vi "Teleop.vi"(10 "Match Info":T1={"Autonomous Elapsed Seconds"=0.0, "TeleOp Elapsed Seconds"=0.0, "Disabled Elapsed Seconds"=0.0, "Visited Autonomous"=FALSE, "Visited TeleOp"=FALSE, "Visited Disabled"=FALSE, "Autonomous Settings"={"Autonomous Style"=enum."Independent", "VI Refnum"=refnum}}, 11 "Call Context":T2) -> ()   [LabVIEW 2017]
doc: "This VI is called for each TeleOp packet received from the DS where the robot is not disabled. It is often used to read from the joysticks and update I/O or to update setpoints for timed control loops. It should complete and return within 20 milliseconds or it may miss DS packets."
uses:
  <vilib>/Rock Robotics/WPI/DriverStation/WPI_DriverStationDerivedRobotMode.ctl
  <vilib>/Rock Robotics/WPI/DriverStation/WPI_DriverStationMatch Info.ctl
  Drive/Drive Notifier.ctl
  Drive/Drive Control Type.ctl
  Intake/Intake Notifier.ctl
  Intake/Intake Control Type.ctl
  Lift/Lift Notifier.ctl
  Lift/Lift Control Type.ctl
  Lift/Lift Enum States.ctl
  RPED/RPED Notifier.ctl
  RPED/RPED Control Type.ctl
  Intake Rotation/Intake Rotation Notifier.ctl
  Intake Rotation/Intake Rotation Control Type.ctl
  Intake Rotation/Arm Enum States.ctl
  LEDs/LED Notifier.ctl
  LEDs/LED Control Type.ctl
  <vilib>/Rock Robotics/Network Tables/NT Write String.vi
  Drive/Drive Globals.vi
  Lift/Lift Globals.vi
  Intake/Intake Globals.vi
  RPED/RPED Globals.vi
  Intake Rotation/Intake Rotation Globals.vi
  LEDs/LED Globals.vi
  Utility VIs/Refnum Names.vi
  <vilib>/Rock Robotics/WPI/Utilities/WPI_GetSetVariantRefNum.vi
  Robot Global Data.vi
panel:
  out "Visited Disabled":bool
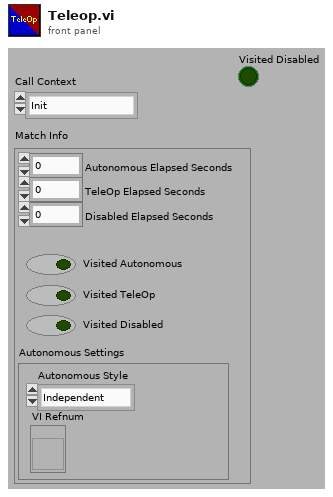
[diagram p1: front panel]
types:
  T1 = typedef "WPI_DriverStationMatch Info.ctl" = cluster{"Autonomous Elapsed Seconds":dbl, "TeleOp Elapsed Seconds":dbl, "Disabled Elapsed Seconds":dbl, "Visited Autonomous":bool, "Visited TeleOp":bool, "Visited Disabled":bool, "Autonomous Settings":cluster{"Autonomous Style":enum16{"Iterative", "Independent"}, "VI Refnum":refnum<vi>}}
  T2 = typedef "WPI_DriverStationDerivedRobotMode.ctl" = enum16{"Init", "Execute", "Stop"}
  T3 = typedef "LED Notifier.ctl" = cluster{"LED Control Type":T4, "Climbing":bool, "Auto Tracking":bool, "Ready for Cube Floor":bool, "Ready for Cube Portal":bool}
  T4 = typedef "LED Control Type.ctl" = enum16{"Off", "Waiting On Field", "Connected ", "Cube In Intake", "Climbing", "Auto Cube Capture", "Ready for Cube Floor", "Ready for Cube Portal"}
  T5 = typedef "Intake Rotation Notifier.ctl" = cluster{"Step":i32, "Intake Rotation Control Type":T6, "Parameter 1":dbl, "Parameter 2":dbl, "Intake Rotation Notifier":refnum<notifier>, "Manual Up":bool, "Manual Down":bool, "Climb":bool, "Switch":bool, "Scale Low":bool, "Scale High":bool, "Stow":bool, "Load":bool, "Scale Mid":bool, "Exchange":bool, "Set Position":T7, "Portal":bool}
  T6 = typedef "Intake Rotation Control Type.ctl" = enum16{"No Op", "Manual Up", "Position", "Manual Down", "PositionAuto"}
  T7 = typedef "Arm Enum States.ctl" = enum16{"Current Position", "Climb", "Load", "Portal", "Switch", "Scale High", "Scale Mid", "Scale Low", "Exchange", "Stow"}
  T8 = typedef "RPED Notifier.ctl" = cluster{"RPED Control Type":T9, "Step":i32, "Left Forward":bool, "Right Forward":bool, "Parameter 1":dbl, "Parameter 2":dbl, "Parameter 3":dbl, "RPED Notifier":refnum<notifier>, "Left Back":bool, "Right Back":bool, "Right":bool, "Left":bool}
  T9 = typedef "RPED Control Type.ctl" = enum16{"No Op", "Left Manual", "Right Manual", "Time", "Left", "Right", "Left_Slow", "Right_Slow", "Left_Distance", "Right_Distance"}
  T10 = typedef "Lift Notifier.ctl" = cluster{"Lift Control Type":T11, "Step":i32, "Set Position":T12, "Climb":bool, "Switch":bool, "Scale Low":bool, "Scale Mid":bool, "Scale High":bool, "Stow":bool, "Load":bool, "Climb Actuation":bool, "Manual Up":bool, "Manual Down":bool, "Parameter 1":dbl, "Parameter 2":dbl, "Parameter 3":dbl, "Lift Notifier":refnum<notifier>, "Exchange":bool, "Brake":bool, "Portal":bool}
  T11 = typedef "Lift Control Type.ctl" = enum16{"No Op", "Position", "Climb Actuation", "Manual Up", "Manual Down", "PositionAuto", "Position_kP", "Position_Delay"}
  T12 = typedef "Lift Enum States.ctl" = enum16{"Climb", "Load", "Portal", "Switch", "Scale High", "Scale Mid", "Scale Low", "Exchange", "Stow", "Current Position"}
  T13 = typedef "Intake Notifier.ctl" = cluster{"Intake Control Type":T14, "Step":i32, "In":bool, "Speed":dbl, "Out":bool, "Parameter 1":dbl, "Parameter 2":dbl, "Intake Notifier":refnum<notifier>, "Actuate Cube":bool, "Speed In":dbl, "Speed Out":dbl, "Load":bool, "Override":bool, "Exchange":bool, "Intake Open":bool}
  T14 = typedef "Intake Control Type.ctl" = enum16{"No Op", "In", "Out", "Test Mode", "Cube_In", "Cube_Out", "State_Change"}
  T15 = typedef "Drive Notifier.ctl" = cluster{"Drive Control Type":T16, "Throttle":dbl, "Twist":dbl, "Step":i32, "High Gear":bool, "Parameter 1":dbl, "Parameter 2":dbl, "Parameter 3":dbl, "Drive Notifier":refnum<notifier>, "AutoTrack":bool}
  T16 = typedef "Drive Control Type.ctl" = enum16{"No_Op", "Basic Drive", "Time", "Heading", "Hybrid_Turn", "RC_Speed", "Switch_Slots", "AutoTrack_Cube", "Speed Test", "Turn_Cube", "To_Cube", "Wait", "Distance_Slow", "Distance", "D_H_Delay", "Distance_Delay", "Heading_Cap", "Heading_Tight", "Cube_Heading", "Distance_Ramp"}
  T17 = typedef "Joystick Controls.ctl" = cluster{"Pilot Left Joystick X":dbl, "Pilot Left Joystick Y":dbl, "Pilot A Button":bool, "Pilot B Button":bool, "Pilot X Button":bool, "Pilot Y Button":bool, "Pilot Left Bumper":bool, "Pilot Right Bumper":bool, "Pilot View Button":bool, "Pilot Menu Button":bool, "Pilot Left Joystick Press":bool, "Pilot Right Joystick Press":bool, "Pilot Left Trigger":dbl, "Pilot Right Joystick X":dbl, "Pilot Right Joystick Y":dbl, "Pilot Right Trigger":dbl, "Copilot Left Joystick X":dbl, "Copilot Left Joystick Y":dbl, "Copilot A Button":bool, "Copilot B Button":bool, "Copilot X Button":bool, "Copilot Y Button":bool, "Copilot Left Bumper":bool, "Copilot Right Bumper":bool, "Copilot View Button":bool, "Copilot Menu Button":bool, "Copilot Left Joystick Press":bool, "Copilot Right Joystick Press":bool, "Copilot Left Trigger":dbl, "Copilot Right Joystick X":dbl, "Copilot Right Joystick Y":dbl, "Copilot Right Trigger":dbl, "Pilot D-Pad":i16, "Copilot D-Pad":i16}
  T18 = typedef "WPI_CompressorDevRef.ctl" = cluster{"DevStatus":errorcluster, "Pneumatics Control Module":u8}
  T19 = cluster{"offsetAngle H":dbl, "offsetAngle V":dbl, "area":dbl, "skew":dbl}
  T20 = typedef "WPI_JoystickDevRef.ctl" = cluster{"Device":T21}
  T21 = typedef "WPI_JoystickDeviceEnum.ctl" = enum16{"USB 0", "USB 1", "USB 2", "USB 3", "USB 4", "USB 5"}
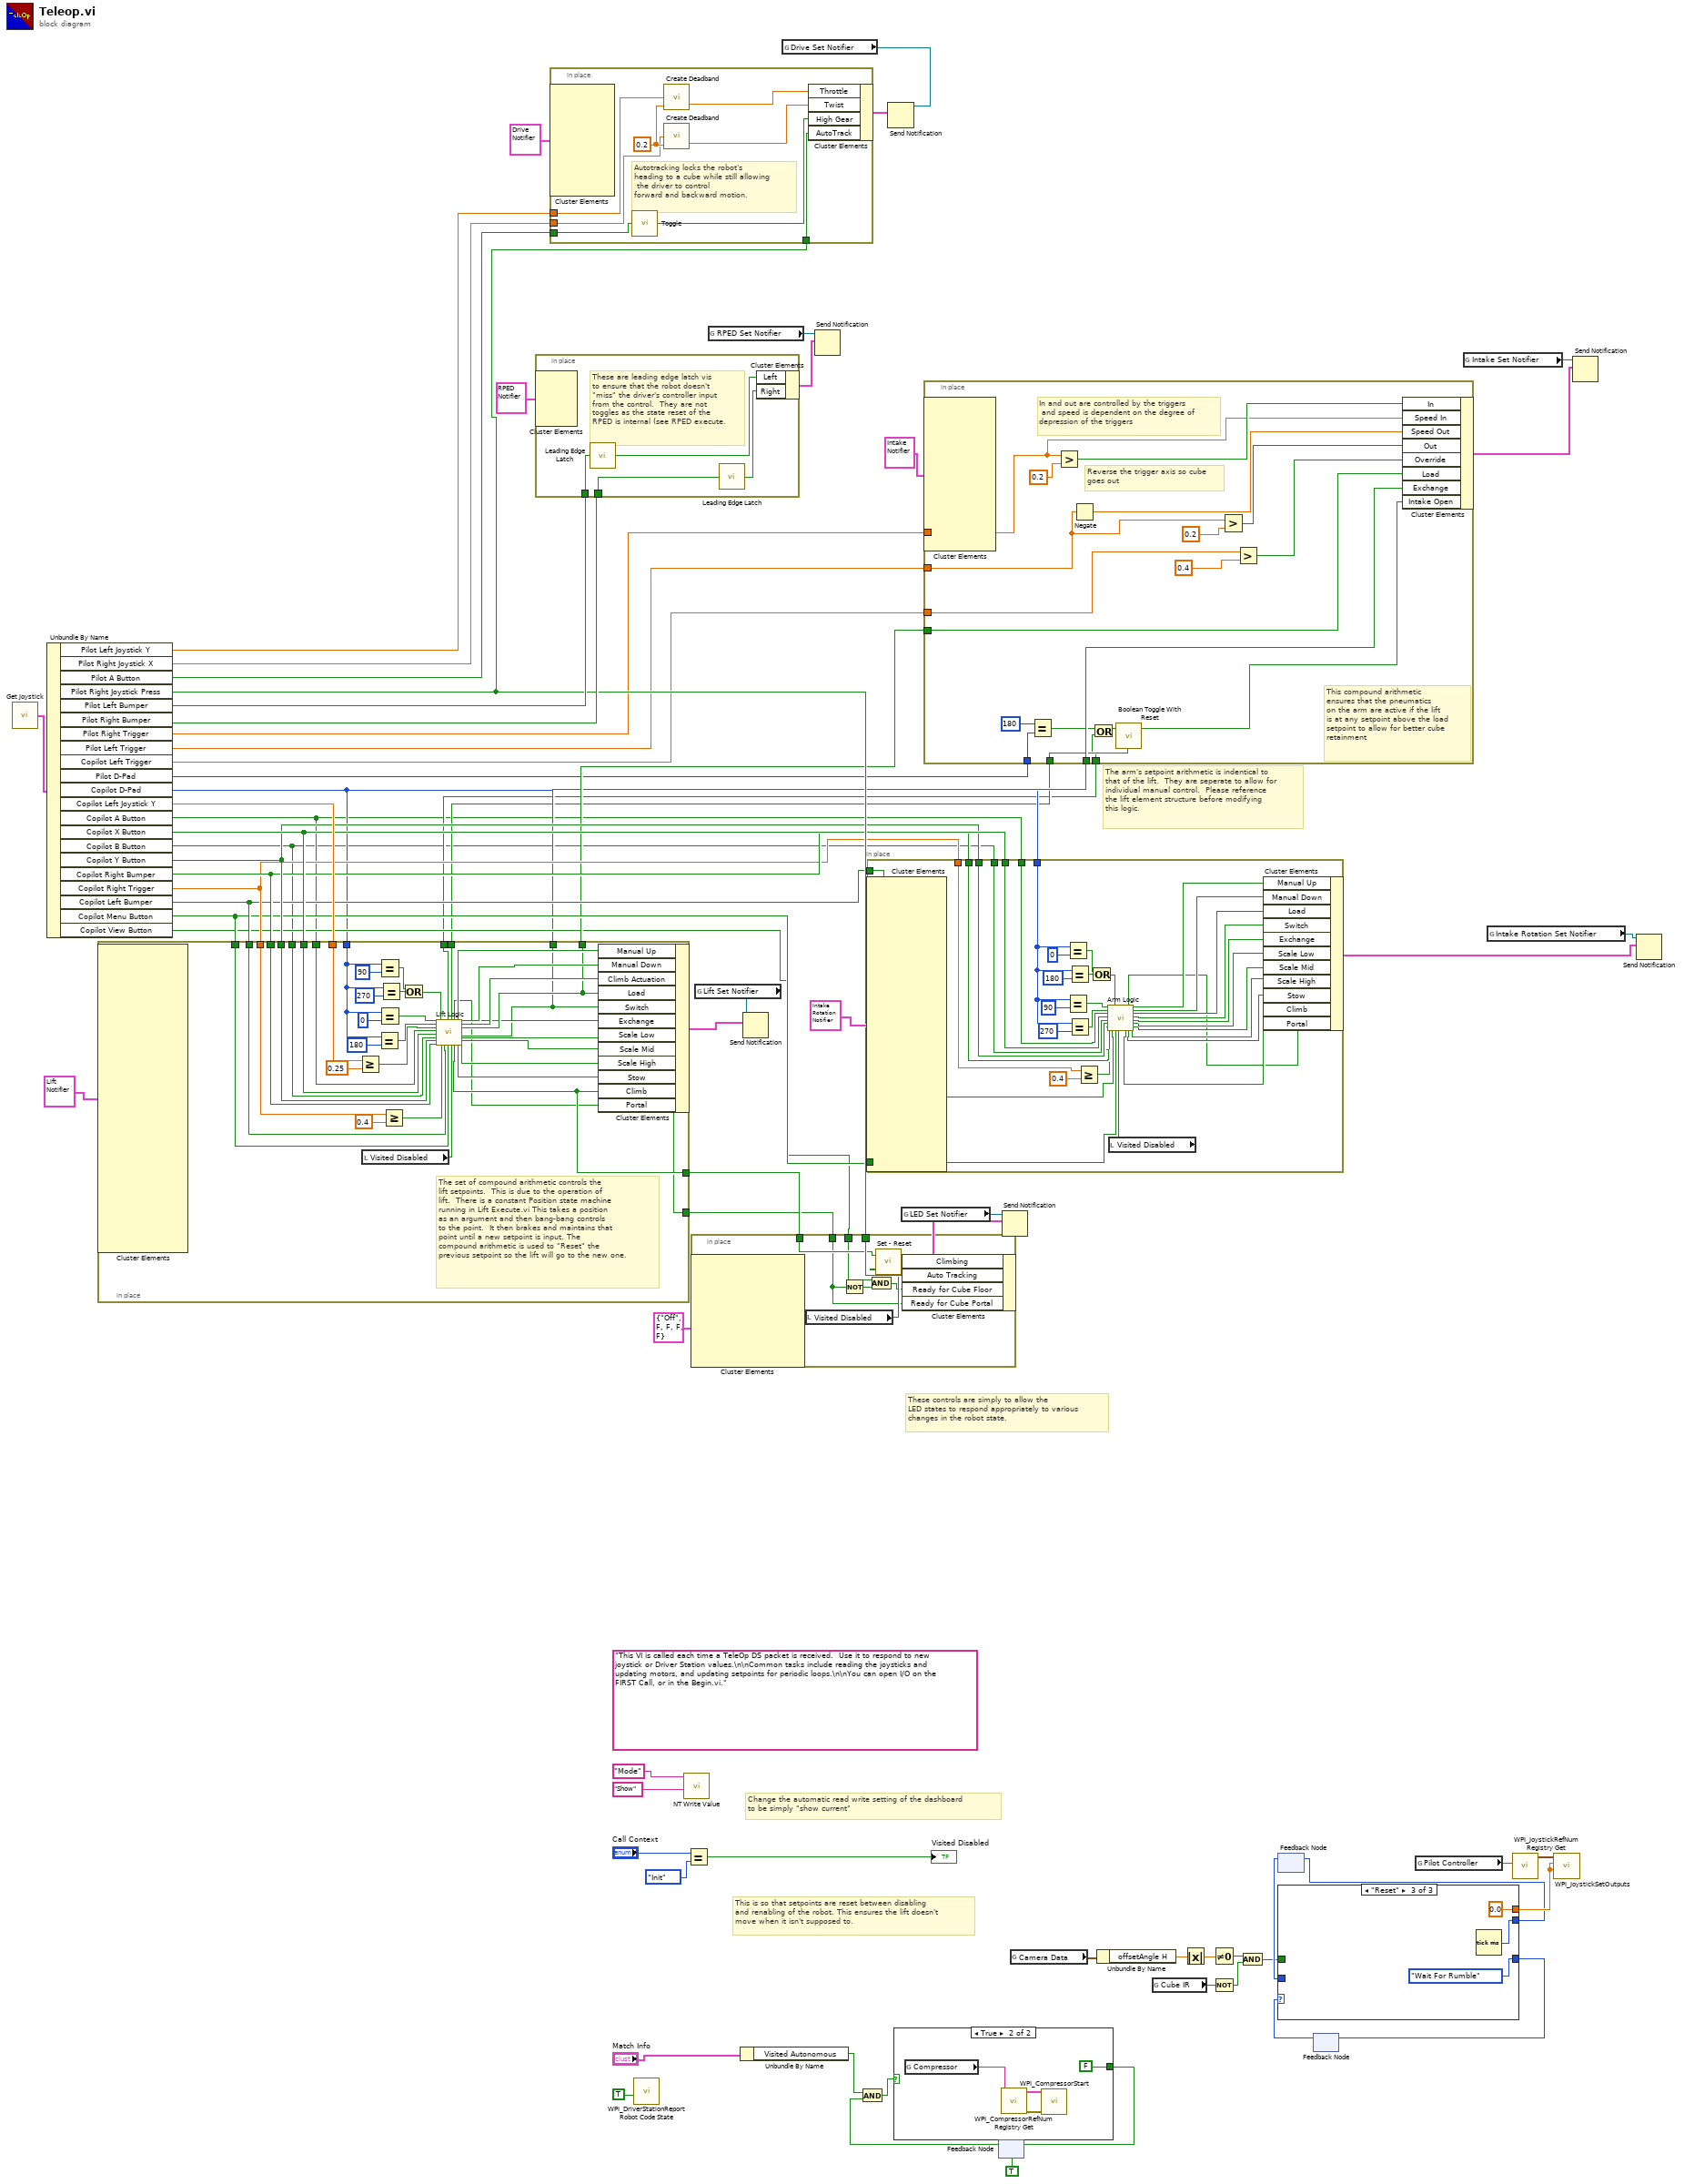
[diagram p0: block diagram]
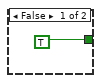
[diagram p2: hidden frame]
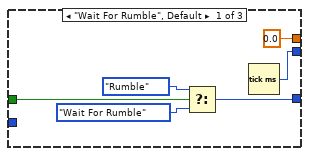
[diagram p3: hidden frame]
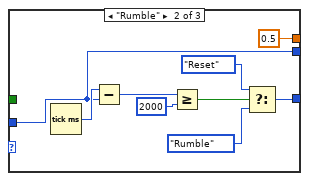
[diagram p4: hidden frame]
diagram:
  (unwired) "This VI is called each time a TeleOp DS packet is received.  Use it to respond to new joystick or Driver Station values.\n\nCommon tasks include reading the joysticks and updating motors, and updating setpoints for periodic loops.\n\nYou can open I/O on the FIRST Call, or in the Begin.vi."
  # "The arm's setpoint arithmetic is indentical to \nthat of the lift.  They are seperate to allow for\nindividual manual control.  Please reference \nthe lift element structure before modifying\nthis logic."
  # "Change the automatic read write setting of the dashboard\nto be simply \"show current\""
  # "This is so that setpoints are reset between disabling\nand renabling of the robot. This ensures the lift doesn't\nmove when it isn't supposed to."
  # "These controls are simply to allow the \nLED states to respond appropriately to various\nchanges in the robot state."
  n1 = call "Get Joystick.vi"() -> ("Joystick Controls"=w71:T17)  [unwired: 7 in]
  n2 = Unbundle By Name(w71) -> ("Pilot Left Joystick Y"=w39:dbl, "Pilot Right Joystick X"=w36:dbl, "Pilot A Button"=w35:bool, "Pilot Right Joystick Press"=w34:bool, "Pilot Left Bumper"=w38:bool, "Pilot Right Bumper"=w37:bool, "Pilot Right Trigger"=w33:dbl, "Pilot Left Trigger"=w32:dbl, "Copilot Left Trigger"=w24:dbl, "Pilot D-Pad"=w6:i16, "Copilot D-Pad"=w7:i16, "Copilot Left Joystick Y"=w31:dbl, "Copilot A Button"=w2:bool, "Copilot X Button"=w30:bool, "Copilot B Button"=w1:bool, "Copilot Y Button"=w29:bool, "Copilot Right Bumper"=w28:bool, "Copilot Right Trigger"=w27:dbl, "Copilot Left Bumper"=w26:bool, "Copilot Menu Button"=w25:bool, "Copilot View Button"=w22:bool)
  n3 = in-place {
    in-place-border: w7 -> [w73]
    in-place-border: w31 -> [w104]
    in-place-border: w2 -> [w102]
    in-place-border: w30 -> [w101]
    in-place-border: w1 -> [w100]
    in-place-border: w29 -> [w99]
    in-place-border: w28 -> [w98]
    in-place-border: w27 -> [w97]
    in-place-border: w26 -> [w85]
    in-place-border: w25 -> [w87]
    in-place-border: [w88] -> w23
    in-place-border: [w86] -> w15
    in-place-border: [w82] -> w14
    in-place-border: [w81] -> w5
    in-place-border: [w80] -> w4
    in-place-border: [w79] -> w3
    # "The set of compound arithmetic controls the \nlift setpoints.  This is due to the operation of \nlift.  There is a constant Position state machine\nrunning in Lift Execute.vi This takes a position\nas an argument and then bang-bang controls\nto the point.  It then brakes and maintains that\npoint until a new setpoint is input. The \ncompound arithmetic is used to \"Reset\" the\nprevious setpoint so the lift will go to the new one."
    n4 = in-place-cluster #1(T10 {"Lift Control Type"=enum."No Op", "Step"=0, "Set Position"=enum."Load", "Climb"=FALSE, "Switch"=FALSE, "Scale Low"=FALSE, "Scale Mid"=FALSE, "Scale High"=FALSE, "Stow"=FALSE, "Load"=FALSE, "Climb Actuation"=FALSE, "Manual Up"=FALSE, "Manual Down"=FALSE, "Parameter 1"=0.0, "Parameter 2"=0.0, "Parameter 3"=0.0, "Lift Notifier"=refnum, "Exchange"=FALSE, "Brake"=FALSE, "Portal"=FALSE} ("Lift Notifier")) -> ()  [unwired: 12 out]
    n5 = Greater Or Equal?(x=w104, y=0.25) -> (x >= y?=w84:bool)
    n6 = local read "Visited Disabled"() -> (w94:bool)
    n7 = Equal?(x=w73, y=i16 180) -> (x = y?=w107:bool)
    n8 = Equal?(x=w73, y=i16 90) -> (x = y?=w77:bool)
    n9 = Equal?(x=w73, y=i16 0) -> (x = y?=w108:bool)
    n10 = Equal?(x=w73, y=i16 270) -> (x = y?=w78:bool)
    n11 = Greater Or Equal?(x=w97, y=0.4) -> (x >= y?=w95:bool)
    n12 = Or(x=w77, y=w78) -> (x .or. y?=w74:bool)
    n13 = call "Lift Logic.vi"("Manual Up"=w108, "Manual Down"=w107, "Climb Actuation"=w84, "Load"=w102, "Switch"=w101, "Exchange"=w100, "Scale Low"=w99, "Scale Mid"=w98, "Reset State Machine"=w74, "Scale High"=w95, "Stow"=w85, "Climb"=w87, "Visited Disabled"=w94) -> ("Open Arms"=w80:bool, "Reset Arm"=w81:bool, "Portal Out"=w79:bool, "Climb Out"=w86:bool, "Manual Up Out"=w93:bool, "Stow Out"=w109:bool, "Manual Down Out"=w92:bool, "Climb Actuation Out"=w110:bool, "Load Out"=w88:bool, "Switch Out"=w83:bool, "Exchange Out"=w82:bool, "Scale Low Out"=w91:bool, "Scale Mid Out"=w90:bool, "Scale High Out"=w89:bool)  [unwired: 1 in]
    n14 = in-place-cluster #1("Manual Up"=w93, "Manual Down"=w92, "Climb Actuation"=w110, "Load"=w88, "Switch"=w83, "Exchange"=w82, "Scale Low"=w91, "Scale Mid"=w90, "Scale High"=w89, "Stow"=w109, "Climb"=w86, "Portal"=w79) -> (w68:T10)
  }
  n15 = in-place {
    in-place-border: w38 -> [w112]
    in-place-border: w37 -> [w111]
    # "These are leading edge latch vis\nto ensure that the robot doesn't\n\"miss\" the driver's controller input\nfrom the control.  They are not\ntoggles as the state reset of the \nRPED is internal (see RPED execute."
    n16 = in-place-cluster #2(T8 {"RPED Control Type"=enum."No Op", "Step"=0, "Left Forward"=FALSE, "Right Forward"=FALSE, "Parameter 1"=0.0, "Parameter 2"=0.0, "Parameter 3"=0.0, "RPED Notifier"=refnum, "Left Back"=FALSE, "Right Back"=FALSE, "Right"=FALSE, "Left"=FALSE} ("RPED Notifier")) -> ()  [unwired: 2 out]
    n17 = call "Leading Edge Latch.vi"("Input"=w112) -> ("Output"=w114:bool)
    n18 = call "Leading Edge Latch.vi"("Input"=w111) -> ("Output"=w113:bool)
    n19 = in-place-cluster #2("Left"=w114, "Right"=w113) -> (w61:T8)
  }
  n20 = in-place {
    in-place-border: w39 -> [w118]
    in-place-border: w36 -> [w117]
    in-place-border: w35 -> [w116]
    in-place-border: w34 -> [w115]
    w119 = 0.2
    # "Autotracking locks the robot's \nheading to a cube while still allowing\n the driver to control \nforward and backward motion."
    n21 = in-place-cluster #3(T15 {"Drive Control Type"=enum."No_Op", "Throttle"=0.0, "Twist"=0.0, "Step"=0, "High Gear"=FALSE, "Parameter 1"=0.0, "Parameter 2"=0.0, "Parameter 3"=0.0, "Drive Notifier"=refnum, "AutoTrack"=FALSE} ("Drive Notifier")) -> ()  [unwired: 4 out]
    n22 = call "Toggle.vi"("Boolean"=w116) -> ("Boolean Out"=w122:bool)
    n23 = call "Create Deadband.vi"("Input Deadband"=w119, "Input"=w118) -> ("Output"=w121:dbl)  [unwired: 2 in]
    n24 = call "Create Deadband.vi"("Input Deadband"=w119, "Input"=w117) -> ("Output"=w120:dbl)  [unwired: 2 in]
    n25 = in-place-cluster #3("Throttle"=w121, "Twist"=w120, "High Gear"=w122, "AutoTrack"=w115) -> (w70:T15)
  }
  n26 = call <vilib>:"WPI_DriverStationReport Robot Code State.vi"("TeleOp"=TRUE ("Autonomous")) -> ()  [unwired: 10 in, 1 out]
  n27 = call-poly <vilib>:"NT Write Value.vi"("String"="Show", "Name"="Mode") -> ()  [unwired: 9 in, 1 out]
  n28 = Equal?(x="Call Context", y=WPI_DriverStationDerivedRobotMode."Init") -> (x = y?=→"Visited Disabled":bool)
  n29 = in-place {
    in-place-border: w34 -> [w130]
    in-place-border: w22 -> [w125]
    in-place-border: w15 -> [w129]
    in-place-border: w3 -> [w123]
    n30 = in-place-cluster #4(T3 {"LED Control Type"=enum."Off", "Climbing"=FALSE, "Auto Tracking"=FALSE, "Ready for Cube Floor"=FALSE, "Ready for Cube Portal"=FALSE} ("LED Notifier")) -> ()  [unwired: 4 out]
    n31 = local read "Visited Disabled"() -> (w127:bool)
    n32 = Not(x=w123) -> (.not. x?=w124:bool)
    n33 = And(x=w125, y=w124) -> (x .and. y?=w126:bool)
    n34 = call "Set - Reset.vi"("Reset"=w127, "Set"=w129) -> ("Output"=w128:bool)
    n35 = in-place-cluster #4("Climbing"=w128, "Auto Tracking"=w130, "Ready for Cube Floor"=w126, "Ready for Cube Portal"=w123) -> (w52:T3)
  }
  n36 = global read "Lift Globals.vi" "Lift Set Notifier"() -> (w64:refnum<notifier>)
  n37 = global read "RPED Globals.vi" "RPED Set Notifier"() -> (w59:refnum<notifier>)
  n38 = Unbundle By Name("Match Info") -> ("Visited Autonomous"=w11:bool)
  n39 = Send Notification(notification=w68, notifier=w64) -> ()  [unwired: 1 in, 2 out]
  n40 = global read "Drive Globals.vi" "Drive Set Notifier"() -> (w66:refnum<notifier>)
  n41 = Send Notification(notification=w61, notifier=w59) -> ()  [unwired: 1 in, 2 out]
  n42 = in-place {
    in-place-border: w7 -> [w133]
    in-place-border: w2 -> [w148]
    in-place-border: w30 -> [w147]
    in-place-border: w1 -> [w146]
    in-place-border: w29 -> [w145]
    in-place-border: w28 -> [w144]
    in-place-border: w27 -> [w141]
    in-place-border: w26 -> [w140]
    in-place-border: w25 -> [w139]
    n43 = in-place-cluster #5(T5 {"Step"=0, "Intake Rotation Control Type"=enum."No Op", "Parameter 1"=0.0, "Parameter 2"=0.0, "Intake Rotation Notifier"=refnum, "Manual Up"=FALSE, "Manual Down"=FALSE, "Climb"=FALSE, "Switch"=FALSE, "Scale Low"=FALSE, "Scale High"=FALSE, "Stow"=FALSE, "Load"=FALSE, "Scale Mid"=FALSE, "Exchange"=FALSE, "Set Position"=enum."Climb", "Portal"=FALSE} ("Intake Rotation Notifier")) -> ()  [unwired: 11 out]
    n44 = Equal?(x=w133, y=i16 0) -> (x = y?=w132:bool)
    n45 = Equal?(x=w133, y=i16 90) -> (x = y?=w152:bool)
    n46 = Equal?(x=w133, y=i16 180) -> (x = y?=w131:bool)
    n47 = Equal?(x=w133, y=i16 270) -> (x = y?=w151:bool)
    n48 = Greater Or Equal?(x=w141, y=0.4) -> (x >= y?=w142:bool)
    n49 = Or(x=w132, y=w131) -> (x .or. y?=w136:bool)
    n50 = local read "Visited Disabled"() -> (w138:bool)
    n51 = call "Arm Logic.vi"("Manual Up"=w152, "Manual Down"=w151, "Load"=w148, "Switch"=w147, "Exchange"=w146, "Scale Low"=w145, "Scale Mid"=w144, "Scale High"=w142, "Stow"=w140, "Reset State Machine"=w136, "Climb"=w139, "Visited Disabled"=w138) -> ("Climb Out"=w154:bool, "Portal Out"=w137:bool, "Stow Out"=w153:bool, "Manual Up Out"=w162:bool, "Manual Down Out"=w161:bool, "Load Out"=w160:bool, "Switch Out"=w159:bool, "Exchange Out"=w158:bool, "Scale Low Out"=w157:bool, "Scale Mid Out"=w156:bool, "Scale High Out"=w155:bool)  [unwired: 5 in]
    n52 = in-place-cluster #5("Manual Up"=w162, "Manual Down"=w161, "Load"=w160, "Switch"=w159, "Exchange"=w158, "Scale Low"=w157, "Scale Mid"=w156, "Scale High"=w155, "Stow"=w153, "Climb"=w154, "Portal"=w137) -> (w56:T5)
  }
  n53 = Send Notification(notification=w70, notifier=w66) -> ()  [unwired: 1 in, 2 out]
  n54 = global read "LED Globals.vi" "LED Set Notifier"() -> (w50:refnum<notifier>)
  n55 = in-place {
    in-place-border: w33 -> [w176]
    in-place-border: w32 -> [w175]
    in-place-border: w24 -> [w173]
    in-place-border: w23 -> [w171]
    in-place-border: w14 -> [w170]
    in-place-border: w6 -> [w168]
    in-place-border: w5 -> [w166]
    in-place-border: w4 -> [w163]
    # "This compound arithmetic\nensures that the pneumatics\non the arm are active if the lift \nis at any setpoint above the load \nsetpoint to allow for better cube\nretainment"
    # "Reverse the trigger axis so cube\ngoes out"
    # "In and out are controlled by the triggers\n and speed is dependent on the degree of\ndepression of the triggers"
    n56 = in-place-cluster #6(T13 {"Intake Control Type"=enum."No Op", "Step"=0, "In"=FALSE, "Speed"=0.0, "Out"=FALSE, "Parameter 1"=0.0, "Parameter 2"=0.0, "Intake Notifier"=refnum, "Actuate Cube"=FALSE, "Speed In"=0.0, "Speed Out"=0.0, "Load"=FALSE, "Override"=FALSE, "Exchange"=FALSE, "Intake Open"=FALSE} ("Intake Notifier")) -> ()  [unwired: 8 out]
    n57 = Equal?(x=i16 180, y=w168) -> (x = y?=w164:bool)
    n58 = Greater?(x=w176, y=0.2) -> (0:w181:bool)
    n59 = Negate(x=w175) -> (-x=w180:dbl)
    n60 = Or(x=w164, y=w163) -> (x .or. y?=w165:bool)
    n61 = call "Boolean Toggle With Reset.vi"("Input"=w165, "Reset"=w166) -> ("Output"=w167:bool)  [unwired: 25 in]
    n62 = Greater?(x=w175, y=0.2) -> (0:w179:bool)
    n63 = Greater?(x=w173, y=0.4) -> (0:w174:bool)
    n64 = in-place-cluster #6("In"=w181, "Speed In"=w176, "Speed Out"=w180, "Out"=w179, "Override"=w174, "Load"=w171, "Exchange"=w170, "Intake Open"=w167) -> (w69:T13)
  }
  n65 = feedback #7(TRUE) -> (w9:bool)
  n66 = And(x=w11, y=w9) -> (x .and. y?=w12:bool)
  n67 = case shown="True" w12 {
    tunnel: [TRUE FALSE] -> w10
    frame False {
    }
    frame True {
      n68 = global read "Refnum Names.vi" "Compressor"() -> (w186:string)
      n69 = call <vilib>:"WPI_CompressorRefNum Registry Get.vi"("refnum name"=w186) -> ("error out"=w184:errorcluster, "CompressorDevRef"=w185:T18)  [unwired: 9 in]
      n70 = call <vilib>:"WPI_CompressorStart.vi"("error in (no error)"=w184, "CompressorDevRef"=w185) -> ()  [unwired: 8 in, 2 out]
    }
  }
  n71 = feedback-in #7(w10) -> ()
  n72 = Send Notification(notification=w52, notifier=w50) -> ()  [unwired: 1 in, 2 out]
  n73 = global read "Robot Global Data.vi" "Camera Data"() -> (w41:T19)
  n74 = Unbundle By Name(w41) -> ("offsetAngle H"=w40:dbl)
  n75 = global read "Intake Globals.vi" "Cube IR"() -> (w47:bool)
  n76 = Absolute Value(x=w40) -> (abs(x)=w49:dbl)
  n77 = Not Equal To 0?(x=w49) -> (x != 0?=w48:bool)
  n78 = Not(x=w47) -> (.not. x?=w46:bool)
  n79 = And(x=w48, y=w46) -> (x .and. y?=w16:bool)
  n80 = feedback #8() -> (w19:u32)  [unwired: 1 in]
  n81 = feedback #9() -> (w17:enum16{"Wait For Rumble", "Rumble", "Reset"})  [unwired: 1 in]
  n82 = case shown="\"Reset\"" w17 {
    tunnel: [0.0 0.5 0.0] -> w21
    tunnel: [w191 w196 w204] -> w20
    tunnel: w19 -> [_ w196 _]
    tunnel: [w188 w195 enum16{"Wait For Rumble", "Rumble", "Reset"}."Wait For Rumble" ("f")] -> w18
    tunnel: w16 -> [w187 _ _]
    frame "Wait For Rumble", Default {
      n83 = Select(t=enum16{"Wait For Rumble", "Rumble", "Reset"}."Rumble" ("Rumble"), s=w187, f=enum16{"Wait For Rumble", "Rumble", "Reset"}."Wait For Rumble") -> (s? t:f=w188:enum16{"Wait For Rumble", "Rumble", "Reset"})
      n84 = Tick Count (ms)() -> (millisecond timer value=w191:u32)
    }
    frame "Rumble" {
      n85 = Tick Count (ms)() -> (millisecond timer value=w200:u32)
      n86 = Subtract(x=w200, y=w196) -> (x-y=w199:u32)
      n87 = Greater Or Equal?(x=w199, y=u32 2000) -> (x >= y?=w197:bool)
      n88 = Select(t=enum16{"Wait For Rumble", "Rumble", "Reset"}."Reset" ("f"), s=w197, f=enum16{"Wait For Rumble", "Rumble", "Reset"}."Rumble") -> (s? t:f=w195:enum16{"Wait For Rumble", "Rumble", "Reset"})
    }
    frame "Reset" {
      n89 = Tick Count (ms)() -> (millisecond timer value=w204:u32)
    }
  }
  n90 = feedback-in #8(w20) -> ()
  n91 = feedback-in #9(w18) -> ()
  n92 = global read "Refnum Names.vi" "Pilot Controller"() -> (w44:string)
  n93 = global read "Intake Globals.vi" "Intake Set Notifier"() -> (w62:refnum<notifier>)
  n94 = global read "Intake Rotation Globals.vi" "Intake Rotation Set Notifier"() -> (w58:refnum<notifier>)
  n95 = call <vilib>:"WPI_JoystickRefNum Registry Get.vi"("refnum name"=w44) -> ("JoystickDevRef"=w45:T20)  [unwired: 9 in, 1 out]
  n96 = call <vilib>:"WPI_JoystickSetOutputs.vi"("Right Rumble"=w21, "Left Rumble"=w21, "JoystickDevRef"=w45) -> ()  [unwired: 7 in, 2 out]
  n97 = Send Notification(notification=w69, notifier=w62) -> ()  [unwired: 1 in, 2 out]
  n98 = Send Notification(notification=w56, notifier=w58) -> ()  [unwired: 1 in, 2 out]
